vi "GetSubscriberConnections.vi"(3 "Err in":path, 4 "Response":T2, 5 "ROS registered":T4={"topic port"=0, "Node"="", "topic"="", "type"="", "node port"=0, "error "={"status"=FALSE, "code"=0, "source"=""}, "Direction"=enum."Node", "APIs"=[], "Update (ms)"=1, "write queue"=1}) -> (0 "Err out":path, 1 "Subscriber Connections":T3(array[cluster]), 2 "Logs out":T1[](array[typedef]))   [LabVIEW 2012]
uses:
  <userlib>/ROSforLV/ROS/Code/SubVIs/_ROSControl.ctl
  <userlib>/ROSforLV/ROS/Code/SubVIs/_ROSDirection.ctl
  <userlib>/ROSforLV/ROS/Code/Console/Servers/ServerSubs/ROSLog.ctl
  <userlib>/ROSforLV/ROS/Code/Console/Servers/ServerSubs/requestTopic.ctl
  <userlib>/ROSforLV/ROS/Code/_ROSDefinition.vi
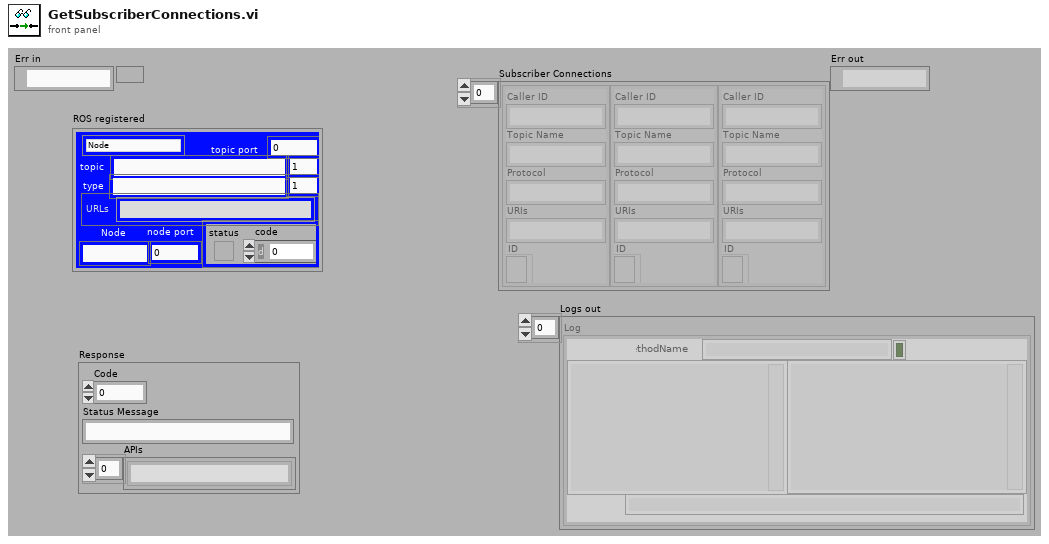
[diagram p1: front panel]
types:
  T1 = typedef "ROSLog.ctl" = cluster{"Sent":string, "Reply":string, "MethodName":string, "success":bool, "Dir1":string, "Dir2":string, "Time Stamp":string, "error":errorcluster, "Preamble":string, "Midamble":string, "Postamble":string}
  T2 = cluster{"Code":i32, "Status Message":string, "APIs":string[]}
  T3 = cluster{"Caller ID":string, "Topic Name":string, "Protocol":string, "URIs":string, "ID":refnum<k5>}[]
  T4 = typedef "_ROSControl.ctl" = cluster{"topic port":u16, "Node":string, "topic":string, "type":string, "node port":u16, "error ":errorcluster, "Direction":T5, "APIs":string[], "Update (ms)":u16, "write queue":u16}
  T5 = typedef "_ROSDirection.ctl" = enum16{"Node", "Publisher", "Subscriber", "Service Client"}
  T6 = typedef "requestTopic.ctl" = cluster{"New Subscriber":cluster{"Caller ID":string, "Topic Name":string, "Protocol":string, "URIs":string, "ID":refnum<k5>}, "ROS of Server":T4, "new port":u16}
  T7 = cluster{"Caller ID":string, "Topic Name":string, "Protocol":string, "URIs":string, "ID":refnum<k5>}
  T8 = cluster{"Protocol":string, "Code":i32, "IP":string, "Port":i32}
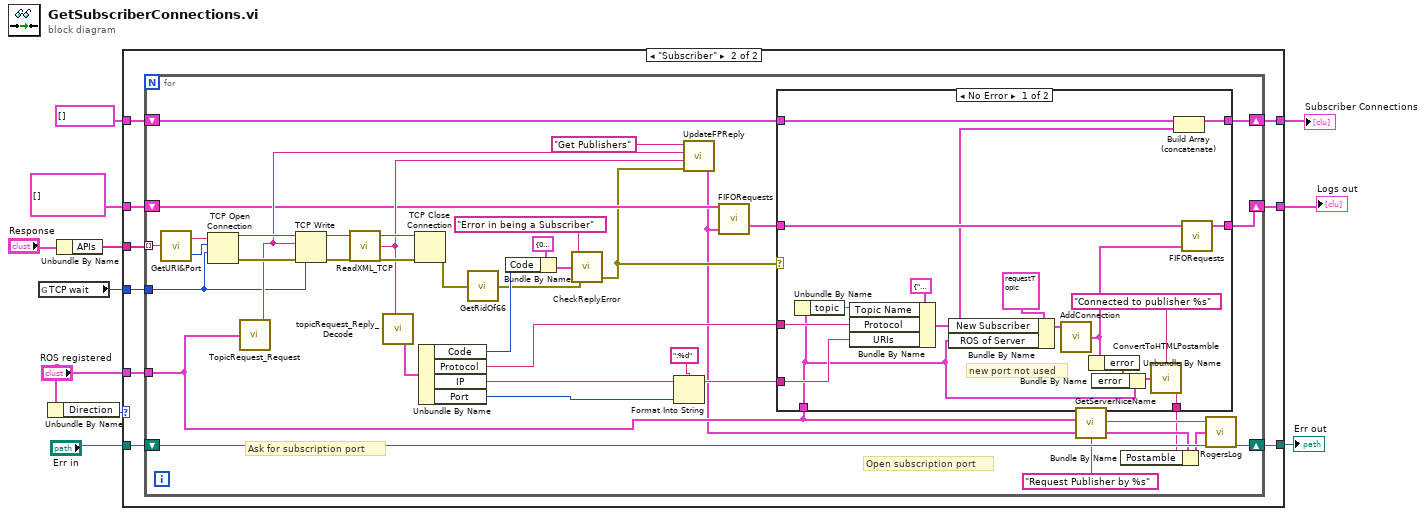
[diagram p0: block diagram]
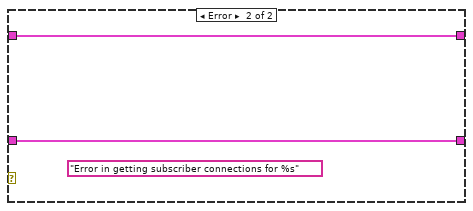
[diagram p3: hidden frame]
diagram:
  n1 = global read "_ROSDefinition.vi" "TCP wait"() -> (w3:i32)
  n2 = Unbundle By Name("ROS registered") -> ("Direction"=w4:T5)
  n3 = Unbundle By Name("Response") -> ("APIs"=w10:string[])
  n4 = case shown="\"Subscriber\"" w4 {
    tunnel: w10 -> [_ w23]
    tunnel: [w14 w22] -> w9
    tunnel: [w13 w21] -> w8
    tunnel: T3 [] ("Subscribers in") -> [w14 w20]
    tunnel: T1[] [] -> [w13 w19]
    tunnel: "ROS registered" -> [_ w18]
    tunnel: w3 -> [_ w17]
    tunnel: "Err in" -> [w12 w16]
    tunnel: [w12 w15] -> w1
    frame Default {
    }
    frame "Subscriber" {
      n5 = for {
        tunnel: w23 -> [w43] mode=indexing
        shift-right: [w41] -> w22
        shift-left: w20 -> [w42]
        shift-right: [w40] -> w21
        shift-left: w19 -> [w36]
        tunnel: w18 -> [w30]
        tunnel: w17 -> [w34]
        shift-right: [w27] -> w15
        shift-left: w16 -> [w31]
        # "Open subscription port"
        # "Ask for subscription port"
        n6 = call <userlib>:"GetURI&Port.vi"("URI in"=w43) -> ("Port"=w62:u16, "URI"=w61:string)
        n7 = TCP Open Connection(address=w61, remote port or service name=w62, timeout ms (60000)=w34) -> (connection ID=w45:refnum<k5>, error out=w44:errorcluster)  [unwired: 2 in]
        n8 = call <userlib>:"TopicRequest_Request.vi"("ROS"=w30) -> ("XML"=w38:string)
        n9 = TCP Write(connection ID=w45, data in=w38, error in (no error)=w44, 9:w34) -> (connection ID out=w46:refnum<k5>, error out=w47:errorcluster)  [unwired: 1 out]
        n10 = call <userlib>:"ReadXML_TCP.vi"("error in"=w47, "connection ID in"=w46) -> ("error out"=w49:errorcluster, "data out"=w37:string, "connection ID out"=w48:refnum<k5>)  [unwired: 1 in]
        n11 = call <userlib>:"topicRequest_Reply_Decode.vi"("Topic Request Reply"=w37) -> ("Topic Request Reply"=w50:T8)
        n12 = TCP Close Connection(connection ID=w48, error in (no error)=w49) -> (error out=w51:errorcluster)  [unwired: 1 in, 1 out]
        n13 = Unbundle By Name(w50) -> ("Code"=w58:i32, "Protocol"=w53:string, "IP"=w55:string, "Port"=w33:i32)
        n14 = call <userlib>:"GetRidOf66.vi"("error in (no error)"=w51) -> ("error out"=w57:errorcluster)
        n15 = Bundle By Name(cluster=T2 {"Code"=0, "Status Message"="", "APIs"=[]} ("Response"), "Code"=w58) -> (w60:T2)
        n16 = call <userlib>:"CheckReplyError.vi"("error in"=w57, "Response"=w60, "Error String"="Error in being a Subscriber" ("source")) -> ("error out"=w32:errorcluster)  [unwired: 2 out]
        n17 = Format Into String(format string=":%d", initial string=w55, w33) -> (resulting string=w54:string)  [unwired: 1 in, 1 out]
        n18 = call <userlib>:"UpdateFPReply.vi"("error in (no error)"=w32, "Reply"=w37, "Sent"=w38, "method"="Get Publishers") -> ("Log"=w26:T1)
        n19 = call <userlib>:"FIFORequests.vi"("Log"=w26, "Requests in"=w36) -> ("Requests out"=w35:T1[])  [unwired: 1 in]
        n20 = case shown="No Error" w32 {
          tunnel: w53 -> [w79 _]
          tunnel: w54 -> [w78 _]
          tunnel: w35 -> [w71 w81]
          tunnel: [w70 w81] -> w40
          tunnel: [w77 w80] -> w41
          tunnel: w30 -> [w64 _]
          tunnel: w42 -> [w76 w80]
          tunnel: [w67 _] -> w24
          frame No Error {
            # "new port not used"
            n21 = Unbundle By Name(w64) -> ("topic"=w74:string)
            n22 = Bundle By Name(cluster=T7 {"Caller ID"="", "Topic Name"="", "Protocol"="", "URIs"="", "ID"=refnum} ("Subscriber"), "Topic Name"=w74, "Protocol"=w79, "URIs"=w78) -> (w69:T7)
            n23 = Bundle By Name(cluster=T6 {"New Subscriber"={"Caller ID"="", "Topic Name"="", "Protocol"="", "URIs"="", "ID"=refnum}, "ROS of Server"={"topic port"=0, "Node"="", "topic"="", "type"="", "node port"=0, "error "={"status"=FALSE, "code"=0, "source"=""}, "Direction"=enum."Node", "APIs"=[], "Update (ms)"=0, "write queue"=0}, "new port"=0} ("data"), "New Subscriber"=w69, "ROS of Server"=w64) -> (w72:T6)
            n24 = call <userlib>:"AddConnection.vi"("data"=w72) -> ("Log"=w66:T1)  [unwired: 3 in, 1 out]
            n25 = Unbundle By Name(w66) -> ("error"=w65:errorcluster)
            n26 = Bundle By Name(cluster=w64, "error"=w65) -> (w63:T4)
            n27 = call <userlib>:"ConvertToHTMLPostamble.vi"("ROS in"=w63, "Text to add"="Connected to publisher %s") -> ("String"=w67:string)
            n28 = Build Array (concatenate)(w76, w69) -> (w77:T3)
            n29 = call <userlib>:"FIFORequests.vi"("Log"=w66, "Requests in"=w71) -> ("Requests out"=w70:T1[])  [unwired: 1 in]
          }
          frame Error {
            (unwired) "Error in getting subscriber connections for %s" ("Error String")
          }
        }
        n30 = call <userlib>:"GetServerNiceName.vi"("ROS"=w30, "Text to add"="Request Publisher by %s") -> ("String"=w28:string)
        n31 = Bundle By Name(cluster=w26, "Postamble"=w24) -> (w25:T1)
        n32 = call <userlib>:"RogersLog.vi"("Text to add"=w28, "Log"=w25, "LogPath in"=w31) -> ("LogPath out"=w27:path)  [unwired: 2 in, 1 out]
      }
    }
  }
  "Subscriber Connections" <- w9
  "Logs out" <- w8
  "Err out" <- w1
